vi "Replace Add Article.vi"(8 "error in (no error)":errorcluster, 9 "Replacement":string, 10 "KEY":string, 11 "Input String":string) -> (0 "error out":errorcluster, 3 "result string":string)   [LabVIEW 2012]
panel:
  out "First letter vowel":bool
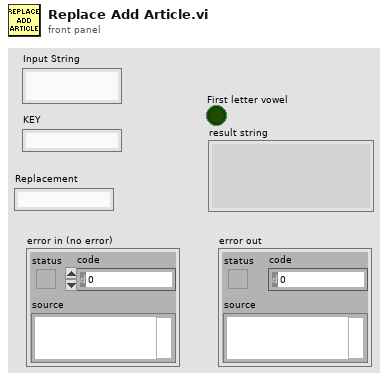
[diagram p1: front panel]
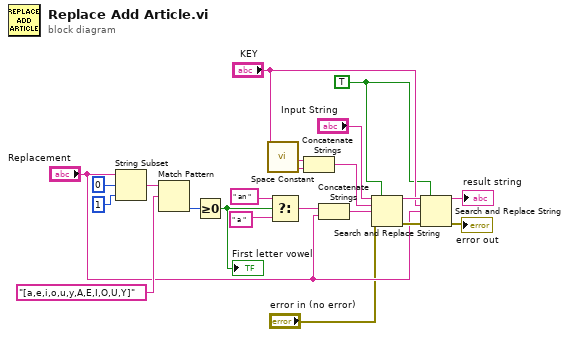
[diagram p0: block diagram]
diagram:
  w3 = TRUE ("replace all? (F)")
  n1 = String Subset(string="Replacement", offset (0)=0, length (rest)=1 ("length (rest)")) -> (substring=w19:string)
  n2 = Match Pattern(string=w19, regular expression="[a,e,i,o,u,y,A,E,I,O,U,Y]") -> (offset past match=w17:i32)  [unwired: 1 in, 3 out]
  n3 = Greater Or Equal To 0?(x=w17) -> (x >= 0?=w13:bool)
  "First letter vowel" <- w13
  n4 = call <vilib>:"Space Constant.vi"() -> ("String"=w15:string)
  n5 = Select(t=" an ", s=w13, f=" a ") -> (s? t:f=w10:string)
  n6 = Concatenate Strings(w15, "KEY") -> (w14:string)
  n7 = Concatenate Strings(w10, "Replacement") -> (w9:string)
  n8 = Search and Replace String(replace all?=w3, input string="Input String", search string=w14, replace string=w9, error in="error in (no error)") -> (result string=w7:string, error out=w8:errorcluster)  [unwired: 3 in, 2 out]
  n9 = Search and Replace String(replace all?=w3, input string=w7, search string="KEY", replace string="Replacement", error in=w8) -> (result string=→"result string":string, error out=→"error out":errorcluster)  [unwired: 3 in, 2 out]
